vi "动态优化.vi"(4 "S_CCw":dbl[](array[numeric]), 5 "S_Cw":dbl[](array[numeric]), 6 "P_CCw":dbl[](array[numeric]), 7 "SENSOR":T1, 8 "P_Cw":dbl[](array[numeric]), 9 "T2_AV(%)":dbl, 10 "T1_AV(%)":dbl) -> (0 "OK？":bool)   [LabVIEW 2020]
uses:
  Global_Variable/Global.vi
  <vilib>/ptbypt/NI_PtbyPt.lvlib
panel:
  in  "initialize 2":bool caption="初始化"
  in  "initialize":bool caption="初始化"
  out "PROC_1":i32
  out "Vres_min_ccw":dbl
  out "Pccw_off(%)":dbl[](array[numeric])
  out "T2ROC1+T2ROC2+T2ROC3":i32
  out "T1ROC1+T1ROC2+T1ROC3":i32
  out "T2ROC_3":i32
  out "T1ROC_3":i32
  out "Pcw_off(%)":dbl[](array[numeric])
  out "Vres_FD":i32
  out "Angle out":dbl
  out "Vres_min_cw":dbl
  out "T2ROC_2":i32
  out "T1ROC_2":i32
  out "PROC":i32
  out "error out":errorcluster caption="错误输出"
  in  "error in (no error)":errorcluster caption="错误输入（无错误）"
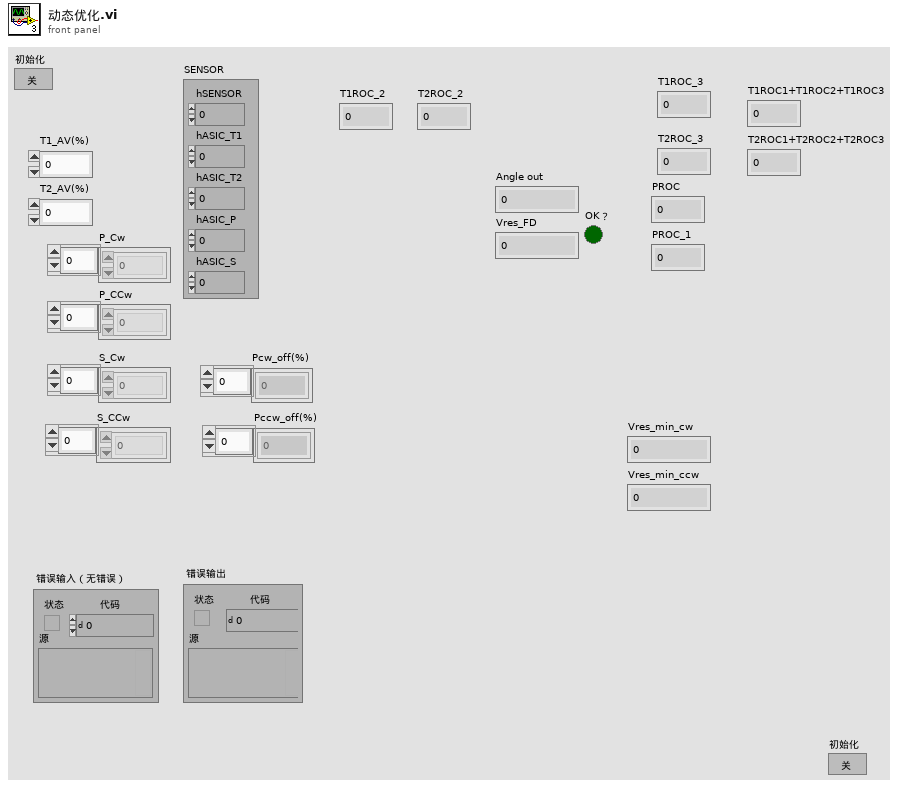
[diagram p1: front panel]
types:
  T1 = cluster{"hSENSOR":i32, "hASIC_T1":i32, "hASIC_T2":i32, "hASIC_P":i32, "hASIC_S":i32}
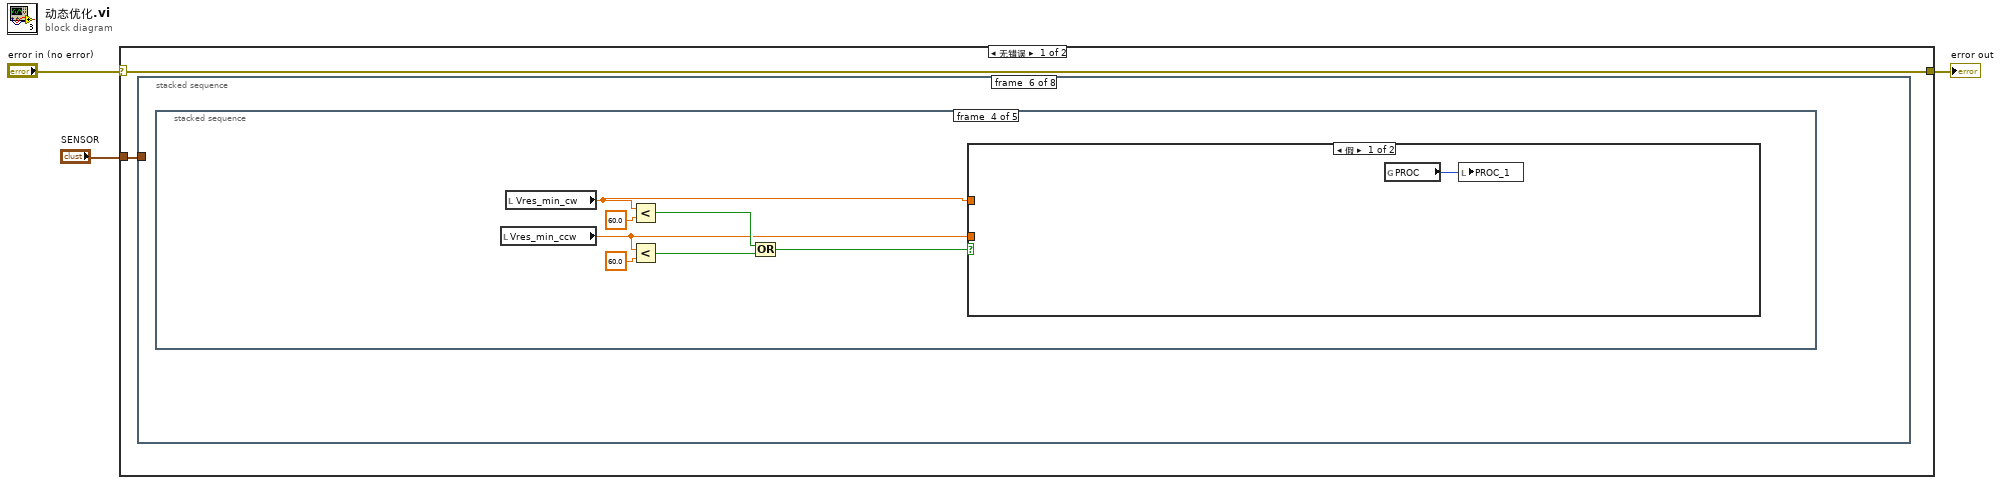
[diagram p0: block diagram]
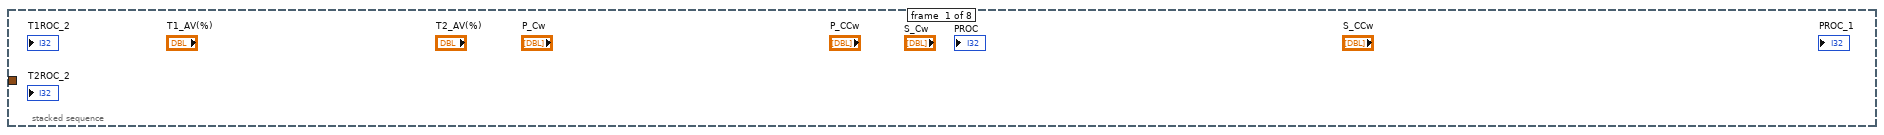
[diagram p2: hidden frame]
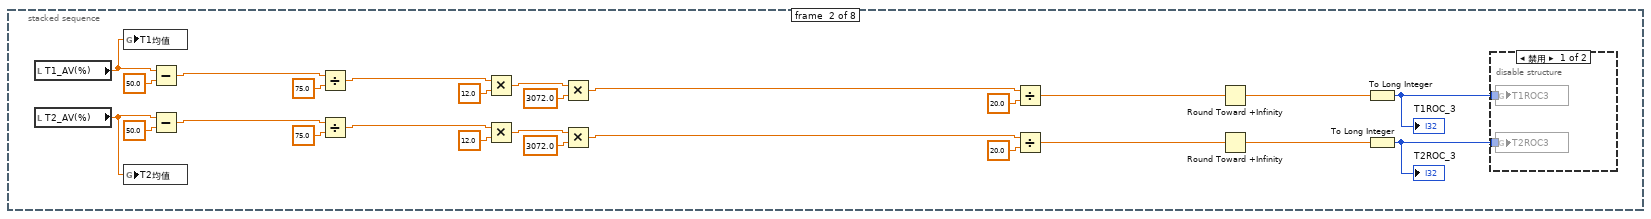
[diagram p3: hidden frame]
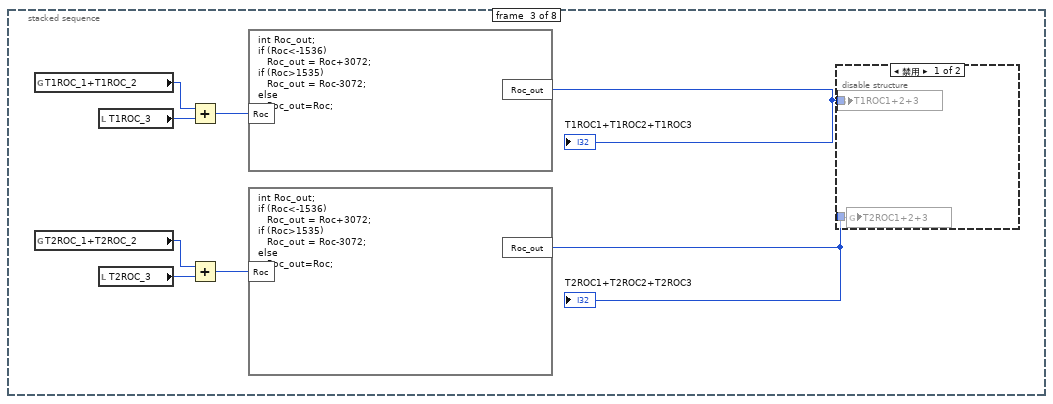
[diagram p5: hidden frame]
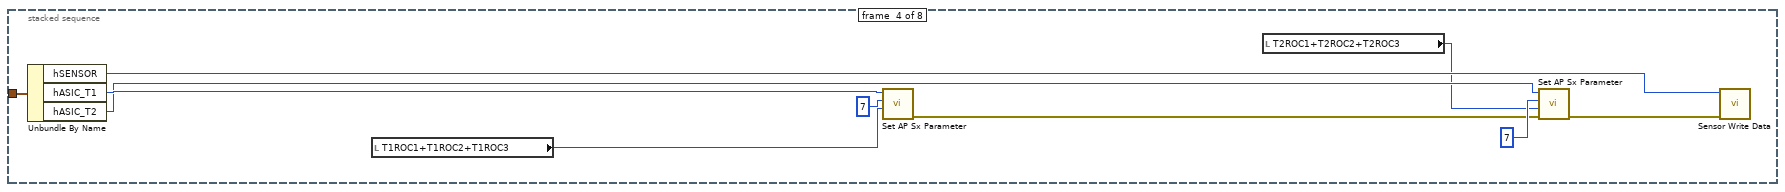
[diagram p7: hidden frame]
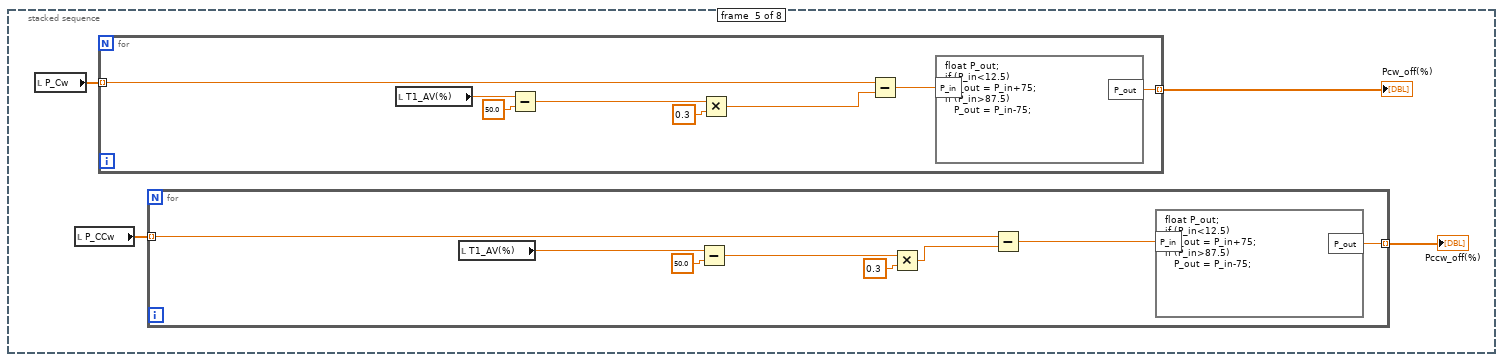
[diagram p8: hidden frame]
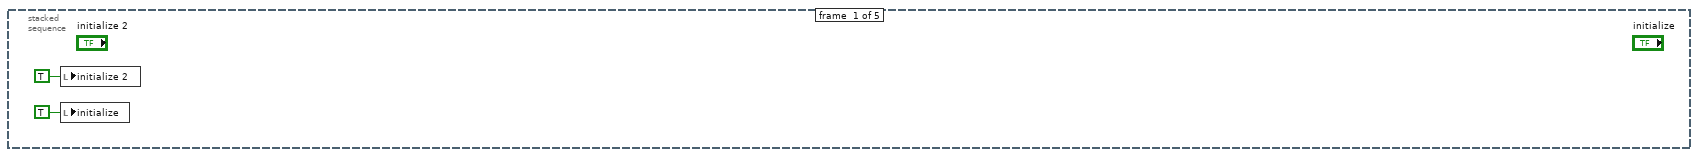
[diagram p9: hidden frame]
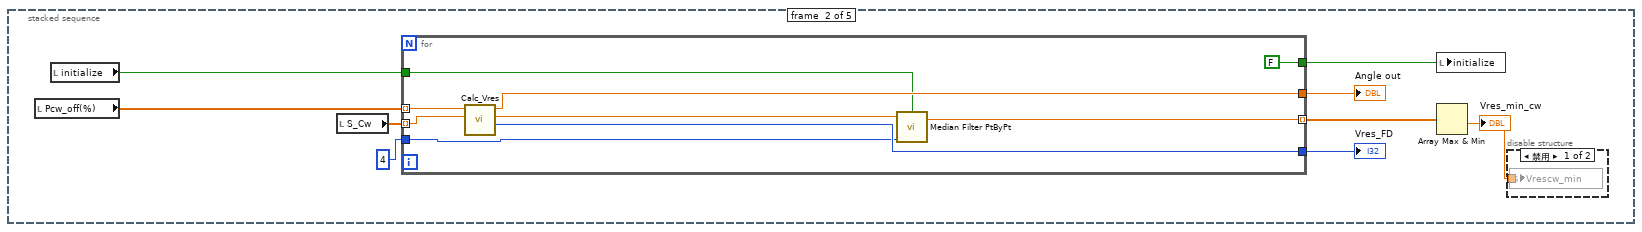
[diagram p10: hidden frame]
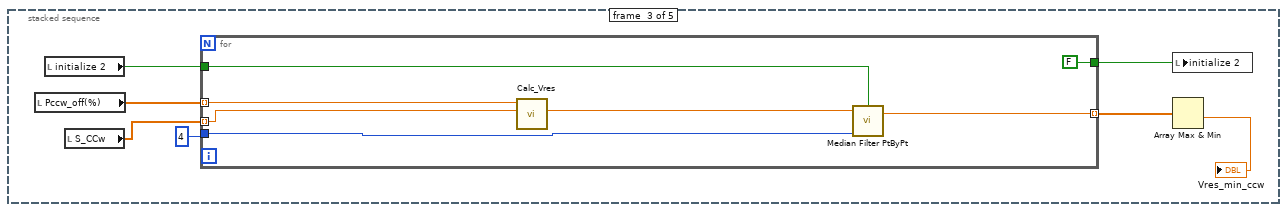
[diagram p12: hidden frame]
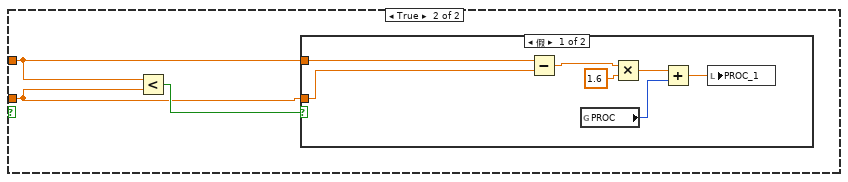
[diagram p13: hidden frame]
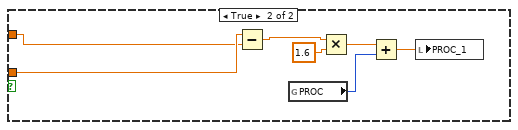
[diagram p14: hidden frame]
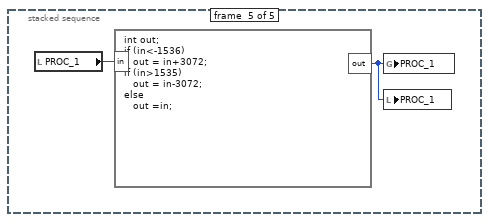
[diagram p15: hidden frame]
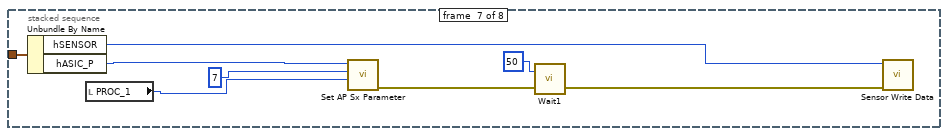
[diagram p16: hidden frame]
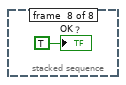
[diagram p17: hidden frame]
diagram:
  n1 = case shown="无错误" "error in (no error)" {
    selector: "error in (no error)" -> [w4 w145]
    tunnel: [w4 w145] -> w2
    tunnel: "SENSOR" -> [w5 _]
    frame No Error {
      n2 = stacked-sequence {
        tunnel: w5 -> [_ _ _ w53 _ _ w143 _]
        frame #0 {
        }
        frame #1 {
          n3 = local read "T1_AV(%)"() -> (w7:dbl)
          n4 = local read "T2_AV(%)"() -> (w6:dbl)
          n5 = global write "Global.vi" "T1均值"(w7) -> ()
          n6 = global write "Global.vi" "T2均值"(w6) -> ()
          n7 = Subtract(x=w7, y=50.0) -> (x-y=w30:dbl)
          n8 = Subtract(x=w6, y=50.0) -> (x-y=w19:dbl)
          n9 = Divide(x=w30, y=75.0) -> (x/y=w28:dbl)
          n10 = Divide(x=w19, y=75.0) -> (x/y=w21:dbl)
          n11 = Multiply(x=w28, y=12.0) -> (x*y=w15:dbl)
          n12 = Multiply(x=w21, y=12.0) -> (x*y=w16:dbl)
          n13 = Multiply(x=w15, y=3072.0) -> (x*y=w13:dbl)
          n14 = Multiply(x=w16, y=3072.0) -> (x*y=w14:dbl)
          n15 = Divide(x=w13, y=20.0) -> (x/y=w17:dbl)
          n16 = Divide(x=w14, y=20.0) -> (x/y=w12:dbl)
          n17 = Round Toward +Infinity(x=w17) -> (ceil(x): smallest int >= x=w10:dbl)
          n18 = Round Toward +Infinity(x=w12) -> (ceil(x): smallest int >= x=w11:dbl)
          n19 = To Long Integer(number=w10) -> (32bit integer=w9:i32)
          "T1ROC_3" <- w9
          n20 = To Long Integer(number=w11) -> (32bit integer=w8:i32)
          "T2ROC_3" <- w8
          n21 = disable-structure shown="禁用" {
            disable-tunnel: w9 -> [w33 _]
            disable-tunnel: w8 -> [w32 _]
            frame Disabled {
              n22 = global write "Global.vi" "T1ROC3"(w33) -> ()
              n23 = global write "Global.vi" "T2ROC3"(w32) -> ()
            }
            frame Enabled {
            }
          }
        }
        frame #2 {
          n24 = global read "Global.vi" "T1ROC_1+T1ROC_2"() -> (w35:i32)
          n25 = global read "Global.vi" "T2ROC_1+T2ROC_2"() -> (w34:i32)
          n26 = local read "T1ROC_3"() -> (w41:i32)
          n27 = local read "T2ROC_3"() -> (w38:i32)
          n28 = Add(x=w35, y=w41) -> (x+y=w40:i32)
          n29 = Add(x=w34, y=w38) -> (x+y=w39:i32)
          n30 = formula code="int Roc_out;\nif (Roc<-1536)\n   Roc_out = Roc+3072;\nif (Roc>1535)\n   Roc_out = Roc-3072;\nelse\n   Roc_out=Roc;"("Roc"=w40) -> ("Roc_out"=w37:i32)
          "T1ROC1+T1ROC2+T1ROC3" <- w37
          n31 = formula code="int Roc_out;\nif (Roc<-1536)\n   Roc_out = Roc+3072;\nif (Roc>1535)\n   Roc_out = Roc-3072;\nelse\n   Roc_out=Roc;"("Roc"=w39) -> ("Roc_out"=w36:i32)
          "T2ROC1+T2ROC2+T2ROC3" <- w36
          n32 = disable-structure shown="禁用" {
            disable-tunnel: w37 -> [w43 _]
            disable-tunnel: w36 -> [w42 _]
            frame Disabled {
              n33 = global write "Global.vi" "T1ROC1+2+3"(w43) -> ()
              n34 = global write "Global.vi" "T2ROC1+2+3"(w42) -> ()
            }
            frame Enabled {
            }
          }
        }
        frame #3 {
          n35 = Unbundle By Name(w53) -> ("hSENSOR"=w50:i32, "hASIC_T1"=w52:i32, "hASIC_T2"=w51:i32)
          n36 = local read "T1ROC1+T1ROC2+T1ROC3"() -> (w45:i32)
          n37 = call "Set AP Sx Parameter.vi"("para2"=w45, "asicBitsName"=7, "asicHandle"=w52) -> ("error out"=w47:errorcluster)  [unwired: 7 in, 1 out]
          n38 = local read "T2ROC1+T2ROC2+T2ROC3"() -> (w44:i32)
          n39 = call "Set AP Sx Parameter.vi"("error in (no error)"=w47, "para2"=w44, "asicBitsName"=7, "asicHandle"=w51) -> ("error out"=w46:errorcluster)  [unwired: 6 in, 1 out]
          n40 = call "Sensor Write Data.vi"("error in (no error)"=w46, "sensorHandle"=w50) -> ()  [unwired: 8 in, 2 out]
        }
        frame #4 {
          n41 = local read "P_Cw"() -> (w57:dbl[])
          n42 = local read "P_CCw"() -> (w54:dbl[])
          n43 = for {
            tunnel: w57 -> [w67] mode=indexing
            tunnel: [w66] -> w56 mode=indexing
            n44 = local read "T1_AV(%)"() -> (w73:dbl)
            n45 = Subtract(x=w73, y=50.0) -> (x-y=w71:dbl)
            n46 = Multiply(x=w71, y=0.3) -> (x*y=w69:dbl)
            n47 = Subtract(x=w67, y=w69) -> (x-y=w68:dbl)
            n48 = formula code="float P_out;\nif (P_in<12.5)\n   P_out = P_in+75;\nif (P_in>87.5)\n   P_out = P_in-75;"("P_in"=w68) -> ("P_out"=w66:dbl)
          }
          "Pcw_off(%)" <- w56
          n49 = for {
            tunnel: w54 -> [w59] mode=indexing
            tunnel: [w58] -> w55 mode=indexing
            n50 = local read "T1_AV(%)"() -> (w65:dbl)
            n51 = Subtract(x=w65, y=50.0) -> (x-y=w63:dbl)
            n52 = Multiply(x=w63, y=0.3) -> (x*y=w61:dbl)
            n53 = Subtract(x=w59, y=w61) -> (x-y=w60:dbl)
            n54 = formula code="float P_out;\nif (P_in<12.5)\n   P_out = P_in+75;\nif (P_in>87.5)\n   P_out = P_in-75;"("P_in"=w60) -> ("P_out"=w58:dbl)
          }
          "Pccw_off(%)" <- w55
        }
        frame #5 {
          n55 = stacked-sequence {
            frame #0 {
              n56 = local write "initialize 2"(TRUE ("initialize 2")) -> ()
              n57 = local write "initialize"(TRUE ("initialize")) -> ()
            }
            frame #1 {
              n58 = local read "Pcw_off(%)"() -> (w83:dbl[])
              n59 = local read "initialize"() -> (w77:bool)
              n60 = local read "S_Cw"() -> (w82:dbl[])
              n61 = for {
                tunnel: [w91] -> w81
                tunnel: [w94] -> w84
                tunnel: w82 -> [w93] mode=indexing
                tunnel: [w89] -> w80 mode=indexing
                tunnel: w83 -> [w92] mode=indexing
                tunnel: 4 ("rank") -> [w88]
                tunnel: w77 -> [w87]
                tunnel: [FALSE ("initialize")] -> w76
                n62 = call "Calc_Vres.vi"("S_Data in"=w93, "P_Data in"=w92) -> ("Vres_FD"=w94:i32, "Vres"=w90:dbl, "Angle out"=w91:dbl)  [unwired: 7 in]
                n63 = call <vilib>:"Median Filter PtByPt.vi"("initialize"=w87, "rank"=w88, "x"=w90) -> ("Filtered x"=w89:dbl)  [unwired: 1 in, 1 out]
              }
              "Angle out" <- w81
              "Vres_FD" <- w84
              n64 = local write "initialize"(w76) -> ()
              n65 = Array Max & Min(array=w80) -> (min value=w79:dbl)  [unwired: 3 out]
              "Vres_min_cw" <- w79
              n66 = disable-structure shown="禁用" {
                disable-tunnel: w79 -> [w85 _]
                frame Disabled {
                  n67 = global write "Global.vi" "Vrescw_min"(w85) -> ()
                }
                frame Enabled {
                }
              }
            }
            frame #2 {
              n68 = local read "Pccw_off(%)"() -> (w101:dbl[])
              n69 = local read "initialize 2"() -> (w96:bool)
              n70 = local read "S_CCw"() -> (w100:dbl[])
              n71 = for {
                tunnel: w100 -> [w108] mode=indexing
                tunnel: [w105] -> w99 mode=indexing
                tunnel: w101 -> [w107] mode=indexing
                tunnel: 4 ("rank") -> [w104]
                tunnel: w96 -> [w103]
                tunnel: [FALSE ("initialize 2")] -> w95
                n72 = call "Calc_Vres.vi"("S_Data in"=w108, "P_Data in"=w107) -> ("Vres"=w106:dbl)  [unwired: 7 in, 2 out]
                n73 = call <vilib>:"Median Filter PtByPt.vi"("initialize"=w103, "rank"=w104, "x"=w106) -> ("Filtered x"=w105:dbl)  [unwired: 1 in, 1 out]
              }
              n74 = local write "initialize 2"(w95) -> ()
              n75 = Array Max & Min(array=w99) -> (min value=→"Vres_min_ccw":dbl)  [unwired: 3 out]
            }
            frame #3 {
              n76 = local read "Vres_min_ccw"() -> (w110:dbl)
              n77 = local read "Vres_min_cw"() -> (w111:dbl)
              n78 = Less?(x=w111, y=60.0) -> (x < y?=w113:bool)
              n79 = Less?(x=w110, y=60.0) -> (x < y?=w112:bool)
              n80 = Or(x=w113, y=w112) -> (x .or. y?=w109:bool)
              n81 = case shown="假" w109 {
                tunnel: w111 -> [_ w118]
                tunnel: w110 -> [_ w117]
                frame False {
                  n82 = global read "Global.vi" "PROC"() -> (w116:i32)
                  n83 = local write "PROC_1"(w116) -> ()
                }
                frame True {
                  n84 = Less?(x=w118, y=w117) -> (x < y?=w119:bool)
                  n85 = case shown="假" w119 {
                    tunnel: w117 -> [w124 w133]
                    tunnel: w118 -> [w125 w132]
                    frame False {
                      n86 = Subtract(x=w125, y=w124) -> (x-y=w126:dbl)
                      n87 = global read "Global.vi" "PROC"() -> (w122:i32)
                      n88 = Multiply(x=w126, y=1.6) -> (x*y=w120:dbl)
                      n89 = Add(x=w120, y=w122) -> (x+y=w121:dbl)
                      n90 = local write "PROC_1"(w121) -> ()
                    }
                    frame True {
                      n91 = Subtract(x=w133, y=w132) -> (x-y=w130:dbl)
                      n92 = global read "Global.vi" "PROC"() -> (w129:i32)
                      n93 = Multiply(x=w130, y=1.6) -> (x*y=w127:dbl)
                      n94 = Add(x=w127, y=w129) -> (x+y=w128:dbl)
                      n95 = local write "PROC_1"(w128) -> ()
                    }
                  }
                }
              }
            }
            frame #4 {
              n96 = local read "PROC_1"() -> (w135:i32)
              n97 = formula code="int out;\nif (in<-1536)\n   out = in+3072;\nif (in>1535)\n   out = in-3072;\nelse\n   out =in;"("in"=w135) -> ("out"=w134:i32)
              n98 = global write "Global.vi" "PROC_1"(w134) -> ()
              n99 = local write "PROC_1"(w134) -> ()
            }
          }
        }
        frame #6 {
          n100 = Unbundle By Name(w143) -> ("hSENSOR"=w141:i32, "hASIC_P"=w142:i32)
          n101 = local read "PROC_1"() -> (w136:i32)
          n102 = call "Set AP Sx Parameter.vi"("para2"=w136, "asicBitsName"=7, "asicHandle"=w142) -> ("error out"=w140:errorcluster)  [unwired: 7 in, 1 out]
          n103 = call "Wait1.vi"("error in (no error)"=w140, "Wait（150ms）"=u32 50) -> ("error out"=w139:errorcluster)  [unwired: 1 in]
          n104 = call "Sensor Write Data.vi"("error in (no error)"=w139, "sensorHandle"=w141) -> ()  [unwired: 8 in, 2 out]
        }
        frame #7 {
          "OK？" <- TRUE ("OK？")
        }
      }
    }
    frame Error {
    }
  }
  "error out" <- w2
